vi "DZ.vi"(1 "Thresh":dbl=0.05 format="%#_13g", 2 "In":dbl) -> (0 "Dz Out":dbl)   [LabVIEW 2013]
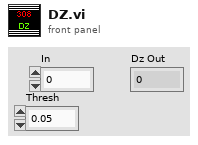
[diagram p1: front panel]
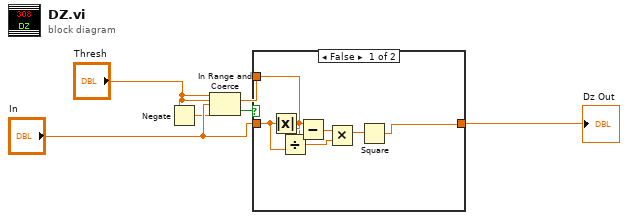
[diagram p0: block diagram]
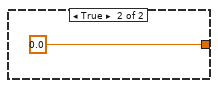
[diagram p2: hidden frame]
diagram:
  n1 = Negate(x="Thresh") -> (-x=w2:dbl)
  n2 = In Range and Coerce(upper limit="Thresh", x="In", lower limit=w2) -> (In Range?=w3:bool)  [unwired: 1 out]
  n3 = case shown="False" w3 {
    tunnel: [w6 0.0] -> w4
    tunnel: "In" -> [w10 _]
    tunnel: "Thresh" -> [w8 _]
    frame False {
      n4 = Absolute Value(x=w10) -> (abs(x)=w11:dbl)
      n5 = Divide(x=w11, y=w10) -> (x/y=w9:dbl)
      n6 = Subtract(x=w11, y=w8) -> (x-y=w12:dbl)
      n7 = Multiply(x=w12, y=w9) -> (x*y=w7:dbl)
      n8 = Square(x=w7) -> (x^2=w6:dbl)
    }
    frame True {
    }
  }
  "Dz Out" <- w4
